vi "cm2nm_maintain_form_values.vi"(1 "Fiducial":bool, 2 "Current Session Information":T1) -> (0 "Cluster":T2)   [LabVIEW 2011]
doc: "Reduce data structure to subset for use with dialog box. Take the old array so we can keep some information for the last entered data."
uses:
  cm2nm_coordinate_information_v2.ctl
  cm2nm_sample_set.ctl
  Instrument_type_enum_v2.ctl
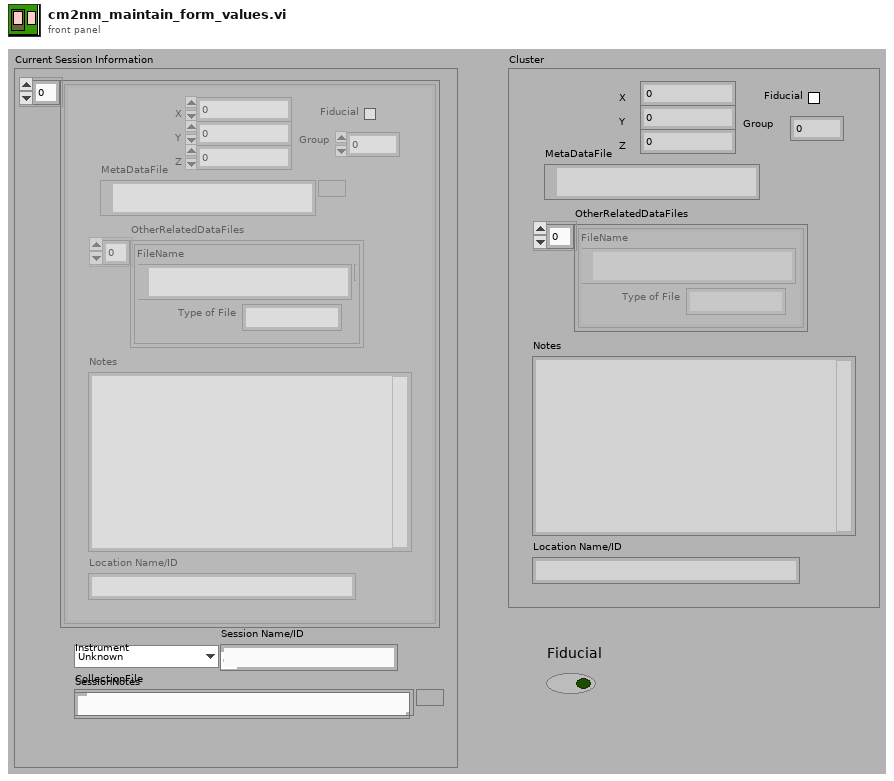
[diagram p1: front panel]
types:
  T1 = typedef "cm2nm_sample_set.ctl" = cluster{"CollectionOfPoints":T2[], "Instrument":T3, "CollectionFile":path, "Session Name/ID":string, "SessionNotes":string}
  T2 = typedef "cm2nm_coordinate_information_v2.ctl" = cluster{"MetaDataFile":path, "X":dbl, "Y":dbl, "Z":dbl, "Group":i32, "Rotation":dbl[unit], "Fiducial":bool, "Magnification":dbl, "Working_Distance":dbl, "Notes":string, "Location Name/ID":string, "OtherRelatedDataFiles":cluster{"Type of File":string, "FileName":path}[], "Available":bool}
  T3 = typedef "Instrument_type_enum_v2.ctl" = enum16{"Unknown", "Philips FEI SEM IRC", "JEOL 7000F EML_MFC", "MXRD MFC", "JEOL_EPMA"}
  T4 = cluster{"Type of File":string, "FileName":path}[]
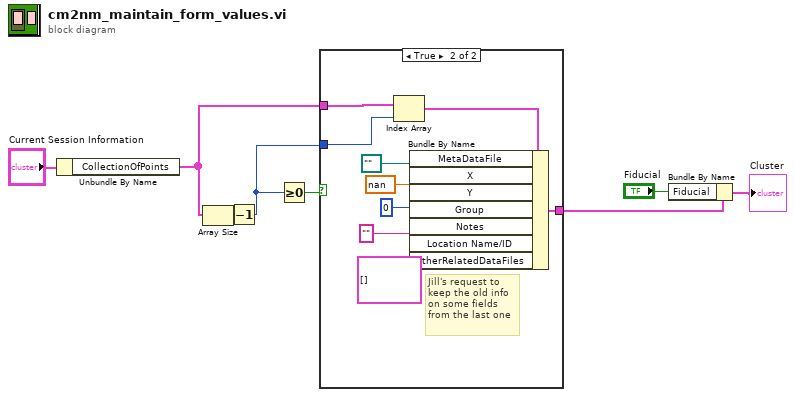
[diagram p0: block diagram]
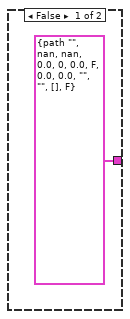
[diagram p2: hidden frame]
diagram:
  n1 = Unbundle By Name("Current Session Information") -> ("CollectionOfPoints"=w4:T2[])
  n2 = Array Size(array=w4) -> (size(s)=w5:i32)
  n3 = Decrement(x=w5) -> (x-1=w8:i32)
  n4 = Greater Or Equal To 0?(x=w8) -> (x >= 0?=w7:bool)
  n5 = case shown="True" w7 {
    tunnel: w4 -> [_ w18]
    tunnel: w8 -> [_ w17]
    tunnel: [T2 {"MetaDataFile"=path "", "X"=nan, "Y"=nan, "Z"=0.0, "Group"=0, "Rotation"=0.0, "Fiducial"=FALSE, "Magnification"=0.0, "Working_Distance"=0.0, "Notes"="", "Location Name/ID"="", "OtherRelatedDataFiles"=[], "Available"=FALSE} ("Cluster") w10] -> w6
    frame False {
    }
    frame True {
      w12 = "" ("Notes")
      w14 = nan ("X")
      # "Jill's request to \nkeep the old info\non some fields\nfrom the last one"
      n6 = Index Array(array=w18, index=w17) -> (element=w16:T2)
      n7 = Bundle By Name(cluster=w16, "MetaDataFile"=path "", "X"=w14, "Y"=w14, "Group"=0, "Notes"=w12, "Location Name/ID"=w12, "OtherRelatedDataFiles"=T4 []) -> (w10:T2)
    }
  }
  n8 = Bundle By Name(cluster=w6, "Fiducial"="Fiducial") -> (→"Cluster":T2)
